vi "robot_position.vi"(10 "Distance Along Arc":u16, 11 "Wheel Angle":i8) -> (1 "New X Position":i16, 2 "New Y Position":i16, 3 "Turning Radius":u8)   [LabVIEW 2009]
uses:
  <vilib>/Platform/TimedLoop/XDataNode/XDataNode.xnode
  <vilib>/Platform/TimedLoop/XDataNode/loadlvalarms.vi
  <vilib>/Platform/TimedLoop/XDataNode/timing_clust.ctl
  <vilib>/Platform/TimedLoop/XDataNode/nitl_modes.ctl
  <vilib>/Platform/TimedLoop/XDataNode/wakeup.ctl
  <vilib>/Platform/TimedLoop/XDataNode/XDNodeRunTimeDep.lvlib
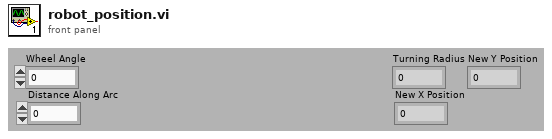
[diagram p1: front panel]
types:
  T1 = typedef "XDNodeRunTimeDep.lvlib/timing_clust.ctl" = cluster{"Expected End [f-1]":u64, "Actual End [f-1]":u64, "Finished Late? [f-1]":bool, "Expected End [i-1]":u64, "Actual End [i-1]":u64, "Finished Late? [i-1]":bool, "Expected Start [i]":u64, "Actual Start [i]":u64, "Expected Start [f]":u64, "Actual Start [f]":u64, "Source Name":string, "Structure Name":string, "Period":i64, "Deadline":i64, "Offset":i64, "Start":i64, "Priority":i32, "Timeout":i32, "Mode":T2, "Wakeup Reason":T3, "Error":errorcluster, "Source Type":string, "Secondary Source Type":string, "Global End Time":u64, "Global Start Time":u64, "Frame Duration":u64, "Iteration Duration":u64, "Assigned CPU":i32, "I/O Scan Engine Mode":u32}
  T2 = typedef "XDNodeRunTimeDep.lvlib/nitl_modes.ctl" = enum32{"No Change", "Process missed periods, maintain original phase", "Discard missed periods, maintain original phase", "Process missed periods, ignore original phase", "Discard missed periods, ignore original phase"}
  T3 = typedef "XDNodeRunTimeDep.lvlib/wakeup.ctl" = enum32{"Normal", "Aborted", "Asynchronous wakeup", "Timing source error", "Timed loop error", "Timeout"}
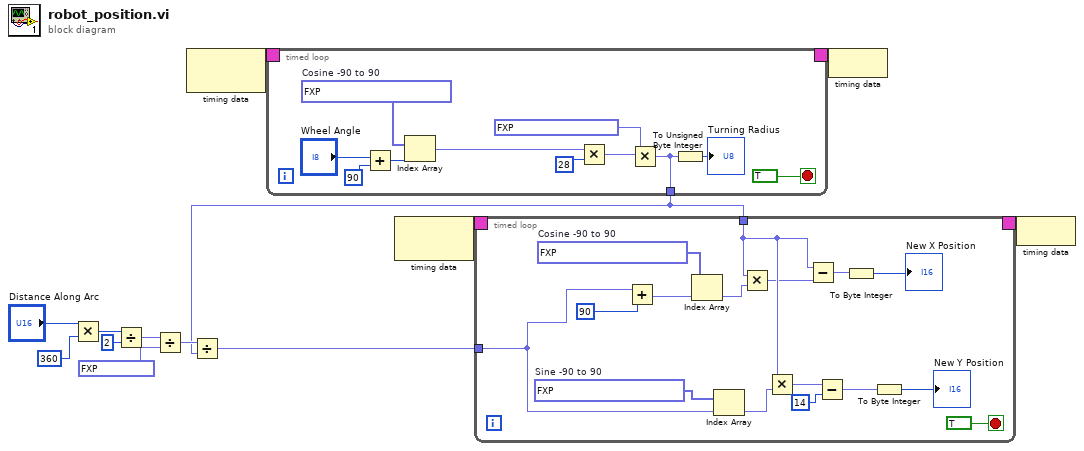
[diagram p0: block diagram]
diagram:
  n1 = Multiply(x="Distance Along Arc", y=u16 360) -> (x*y=w11:u16)
  n2 = Divide(x=w11, y=u8 2) -> (x/y=w6:fxp<+/-,32,16>)
  n3 = Divide(x=w6, y=fxp<+,12,2> 3.1416015625) -> (x/y=w8:fxp<+/-,33,15>)
  n4 = node-c288() -> (w5:T1)  [unwired: 1 in]
  n5 = timed-loop {
    timing: w5 -> [_]
    timing-out: [_] -> w4
    tunnel: [w24] -> w1
    stop <- TRUE stop-if-true
    w22 = fxp<+/-,16,1>[] [0.0, 0.0174560546875, 0.034912109375, 0.052337646484375, 0.06976318359375, 0.087158203125, 0.104522705078125, 0.121856689453125, 0.13916015625, 0.15643310546875, 0.17364501953125, 0.1907958984375, 0.207916259765625, 0.224945068359375, 0.241912841796875, 0.258819580078125, 0.275634765625, 0.2923583984375, 0.30902099609375, 0.3255615234375, 0.342010498046875, 0.358367919921875, 0.374603271484375, 0.390716552734375, 0.40673828125, 0.422607421875, 0.438385009765625, 0.4539794921875, 0.469482421875, 0.48480224609375, 0.5, 0.515045166015625, 0.5299072265625, 0.544647216796875, 0.5592041015625, 0.573577880859375, 0.587799072265625, 0.601806640625, 0.61566162109375, 0.62933349609375, 0.642791748046875, 0.65606689453125, 0.66912841796875, 0.6820068359375, 0.694671630859375, 0.70709228515625, 0.719329833984375, 0.731353759765625, 0.743133544921875, 0.75469970703125, 0.76605224609375, 0.77716064453125, 0.78802490234375, 0.79864501953125, 0.80902099609375, 0.81915283203125, 0.82904052734375, 0.83868408203125, 0.848052978515625, 0.857177734375, 0.86602783203125, 0.8746337890625, 0.8829345703125, 0.891021728515625, 0.8988037109375, 0.90631103515625, 0.913543701171875, 0.920501708984375, 0.92718505859375, 0.93359375, 0.939697265625, 0.945526123046875, 0.9510498046875, 0.956298828125, 0.961273193359375, 0.965911865234375, 0.970306396484375, 0.974365234375, 0.9781494140625, 0.98162841796875, 0.98480224609375, 0.987701416015625, 0.990264892578125, 0.9925537109375, 0.9945068359375, 0.996185302734375, 0.99755859375, 0.998626708984375, 0.9993896484375, 0.999847412109375, 0.999969482421875, 0.999847412109375, 0.9993896484375, 0.998626708984375, 0.99755859375, 0.996185302734375, 0.9945068359375, 0.9925537109375, 0.990264892578125, 0.987701416015625, 0.98480224609375, 0.98162841796875, 0.9781494140625, 0.974365234375, 0.970306396484375, 0.965911865234375, 0.961273193359375, 0.956298828125, 0.9510498046875, 0.945526123046875, 0.939697265625, 0.93359375, 0.92718505859375, 0.920501708984375, 0.913543701171875, 0.90631103515625, 0.8988037109375, 0.891021728515625, 0.8829345703125, 0.8746337890625, 0.86602783203125, 0.857177734375, 0.848052978515625, 0.83868408203125, 0.82904052734375, 0.81915283203125, 0.80902099609375, 0.79864501953125, 0.78802490234375, 0.77716064453125, 0.76605224609375, 0.75469970703125, 0.743133544921875, 0.731353759765625, 0.719329833984375, 0.70709228515625, 0.694671630859375, 0.6820068359375, 0.66912841796875, 0.65606689453125, 0.642791748046875, 0.62933349609375, 0.61566162109375, 0.601806640625, 0.587799072265625, 0.573577880859375, 0.5592041015625, 0.544647216796875, 0.5299072265625, 0.515045166015625, 0.5, 0.48480224609375, 0.469482421875, 0.4539794921875, 0.438385009765625, 0.422607421875, 0.40673828125, 0.390716552734375, 0.374603271484375, 0.358367919921875, 0.342010498046875, 0.3255615234375, 0.30902099609375, 0.2923583984375, 0.275634765625, 0.258819580078125, 0.241912841796875, 0.224945068359375, 0.207916259765625, 0.1907958984375, 0.17364501953125, 0.15643310546875, 0.13916015625, 0.121856689453125, 0.104522705078125, 0.087158203125, 0.06976318359375, 0.052337646484375, 0.034912109375, 0.0174560546875, 0.0]  # Cosine -90 to 90
    n6 = Add(x="Wheel Angle", y=i8 90) -> (x+y=w18:i8)
    n7 = Index Array(array=w22, index=w18) -> (element=w21:fxp<+/-,16,1>)
    n8 = Multiply(x=w21, y=i8 28) -> (x*y=w23:fxp<+/-,24,9>)
    n9 = Multiply(x=w23, y=fxp<+/-,24,9> 3.1416015625) -> (x*y=w24:fxp<+/-,46,16>)
    n10 = To Unsigned Byte Integer(number=w24) -> (unsigned 8bit integer=→"Turning Radius":u8)
  }
  n11 = Divide(x=w8, y=w1) -> (x/y=w7:fxp<+/-,64,45>)
  n12 = node-c288() -> (w3:T1)  [unwired: 1 in]
  n13 = timed-loop {
    timing: w3 -> [_]
    timing-out: [_] -> w2
    tunnel: w7 -> [w42]
    tunnel: w1 -> [w41]
    stop <- TRUE stop-if-true
    w38 = fxp<+/-,16,1>[] [0.0, 0.0174560546875, 0.034912109375, 0.052337646484375, 0.06976318359375, 0.087158203125, 0.104522705078125, 0.121856689453125, 0.13916015625, 0.15643310546875, 0.17364501953125, 0.1907958984375, 0.207916259765625, 0.224945068359375, 0.241912841796875, 0.258819580078125, 0.275634765625, 0.2923583984375, 0.30902099609375, 0.3255615234375, 0.342010498046875, 0.358367919921875, 0.374603271484375, 0.390716552734375, 0.40673828125, 0.422607421875, 0.438385009765625, 0.4539794921875, 0.469482421875, 0.48480224609375, 0.5, 0.515045166015625, 0.5299072265625, 0.544647216796875, 0.5592041015625, 0.573577880859375, 0.587799072265625, 0.601806640625, 0.61566162109375, 0.62933349609375, 0.642791748046875, 0.65606689453125, 0.66912841796875, 0.6820068359375, 0.694671630859375, 0.70709228515625, 0.719329833984375, 0.731353759765625, 0.743133544921875, 0.75469970703125, 0.76605224609375, 0.77716064453125, 0.78802490234375, 0.79864501953125, 0.80902099609375, 0.81915283203125, 0.82904052734375, 0.83868408203125, 0.848052978515625, 0.857177734375, 0.86602783203125, 0.8746337890625, 0.8829345703125, 0.891021728515625, 0.8988037109375, 0.90631103515625, 0.913543701171875, 0.920501708984375, 0.92718505859375, 0.93359375, 0.939697265625, 0.945526123046875, 0.9510498046875, 0.956298828125, 0.961273193359375, 0.965911865234375, 0.970306396484375, 0.974365234375, 0.9781494140625, 0.98162841796875, 0.98480224609375, 0.987701416015625, 0.990264892578125, 0.9925537109375, 0.9945068359375, 0.996185302734375, 0.99755859375, 0.998626708984375, 0.9993896484375, 0.999847412109375, 0.999969482421875, 0.999847412109375, 0.9993896484375, 0.998626708984375, 0.99755859375, 0.996185302734375, 0.9945068359375, 0.9925537109375, 0.990264892578125, 0.987701416015625, 0.98480224609375, 0.98162841796875, 0.9781494140625, 0.974365234375, 0.970306396484375, 0.965911865234375, 0.961273193359375, 0.956298828125, 0.9510498046875, 0.945526123046875, 0.939697265625, 0.93359375, 0.92718505859375, 0.920501708984375, 0.913543701171875, 0.90631103515625, 0.8988037109375, 0.891021728515625, 0.8829345703125, 0.8746337890625, 0.86602783203125, 0.857177734375, 0.848052978515625, 0.83868408203125, 0.82904052734375, 0.81915283203125, 0.80902099609375, 0.79864501953125, 0.78802490234375, 0.77716064453125, 0.76605224609375, 0.75469970703125, 0.743133544921875, 0.731353759765625, 0.719329833984375, 0.70709228515625, 0.694671630859375, 0.6820068359375, 0.66912841796875, 0.65606689453125, 0.642791748046875, 0.62933349609375, 0.61566162109375, 0.601806640625, 0.587799072265625, 0.573577880859375, 0.5592041015625, 0.544647216796875, 0.5299072265625, 0.515045166015625, 0.5, 0.48480224609375, 0.469482421875, 0.4539794921875, 0.438385009765625, 0.422607421875, 0.40673828125, 0.390716552734375, 0.374603271484375, 0.358367919921875, 0.342010498046875, 0.3255615234375, 0.30902099609375, 0.2923583984375, 0.275634765625, 0.258819580078125, 0.241912841796875, 0.224945068359375, 0.207916259765625, 0.1907958984375, 0.17364501953125, 0.15643310546875, 0.13916015625, 0.121856689453125, 0.104522705078125, 0.087158203125, 0.06976318359375, 0.052337646484375, 0.034912109375, 0.0174560546875, 0.0]  # Cosine -90 to 90
    w35 = fxp<+/-,16,1>[] [-1.0, -0.999847412109375, -0.9993896484375, -0.998626708984375, -0.99755859375, -0.996185302734375, -0.9945068359375, -0.9925537109375, -0.990264892578125, -0.987701416015625, -0.98480224609375, -0.98162841796875, -0.9781494140625, -0.974365234375, -0.970306396484375, -0.965911865234375, -0.961273193359375, -0.956298828125, -0.9510498046875, -0.945526123046875, -0.939697265625, -0.93359375, -0.92718505859375, -0.920501708984375, -0.913543701171875, -0.90631103515625, -0.8988037109375, -0.891021728515625, -0.8829345703125, -0.8746337890625, -0.86602783203125, -0.857177734375, -0.848052978515625, -0.83868408203125, -0.82904052734375, -0.81915283203125, -0.80902099609375, -0.79864501953125, -0.78802490234375, -0.77716064453125, -0.76605224609375, -0.75469970703125, -0.743133544921875, -0.731353759765625, -0.719329833984375, -0.70709228515625, -0.694671630859375, -0.6820068359375, -0.66912841796875, -0.65606689453125, -0.642791748046875, -0.62933349609375, -0.61566162109375, -0.601806640625, -0.587799072265625, -0.573577880859375, -0.5592041015625, -0.544647216796875, -0.5299072265625, -0.515045166015625, -0.5, -0.48480224609375, -0.469482421875, -0.4539794921875, -0.438385009765625, -0.422607421875, -0.40673828125, -0.390716552734375, -0.374603271484375, -0.358367919921875, -0.342010498046875, -0.3255615234375, -0.30902099609375, -0.2923583984375, -0.275634765625, -0.258819580078125, -0.241912841796875, -0.224945068359375, -0.207916259765625, -0.1907958984375, -0.17364501953125, -0.15643310546875, -0.13916015625, -0.121856689453125, -0.104522705078125, -0.087158203125, -0.06976318359375, -0.052337646484375, -0.034912109375, -0.0174560546875, 0.0, 0.0174560546875, 0.034912109375, 0.052337646484375, 0.06976318359375, 0.087158203125, 0.104522705078125, 0.121856689453125, 0.13916015625, 0.15643310546875, 0.17364501953125, 0.1907958984375, 0.207916259765625, 0.224945068359375, 0.241912841796875, 0.258819580078125, 0.275634765625, 0.2923583984375, 0.30902099609375, 0.3255615234375, 0.342010498046875, 0.358367919921875, 0.374603271484375, 0.390716552734375, 0.40673828125, 0.422607421875, 0.438385009765625, 0.4539794921875, 0.469482421875, 0.48480224609375, 0.5, 0.515045166015625, 0.5299072265625, 0.544647216796875, 0.5592041015625, 0.573577880859375, 0.587799072265625, 0.601806640625, 0.61566162109375, 0.62933349609375, 0.642791748046875, 0.65606689453125, 0.66912841796875, 0.6820068359375, 0.694671630859375, 0.70709228515625, 0.719329833984375, 0.731353759765625, 0.743133544921875, 0.75469970703125, 0.76605224609375, 0.77716064453125, 0.78802490234375, 0.79864501953125, 0.80902099609375, 0.81915283203125, 0.82904052734375, 0.83868408203125, 0.848052978515625, 0.857177734375, 0.86602783203125, 0.8746337890625, 0.8829345703125, 0.891021728515625, 0.8988037109375, 0.90631103515625, 0.913543701171875, 0.920501708984375, 0.92718505859375, 0.93359375, 0.939697265625, 0.945526123046875, 0.9510498046875, 0.956298828125, 0.961273193359375, 0.965911865234375, 0.970306396484375, 0.974365234375, 0.9781494140625, 0.98162841796875, 0.98480224609375, 0.987701416015625, 0.990264892578125, 0.9925537109375, 0.9945068359375, 0.996185302734375, 0.99755859375, 0.998626708984375, 0.9993896484375, 0.999847412109375, 0.999969482421875]  # Sine -90 to 90
    n14 = Add(x=w42, y=u16 90) -> (x+y=w39:fxp<+/-,64,46>)
    n15 = Index Array(array=w38, index=w39) -> (element=w37:fxp<+/-,16,1>)
    n16 = Index Array(array=w35, index=w42) -> (element=w34:fxp<+/-,16,1>)
    n17 = Multiply(x=w41, y=w37) -> (x*y=w36:fxp<+/-,60,15>)
    n18 = Multiply(x=w41, y=w34) -> (x*y=w33:fxp<+/-,60,15>)
    n19 = Subtract(x=w41, y=w36) -> (x-y=w31:fxp<+/-,62,17>)
    n20 = Subtract(x=w33, y=i8 14) -> (x-y=w29:fxp<+/-,61,16>)
    n21 = To Byte Integer(number=w31) -> (8bit integer=→"New X Position":i8)
    n22 = To Byte Integer(number=w29) -> (8bit integer=→"New Y Position":i8)
  }
  n23 = node-c288(w4) -> ()
  n24 = node-c288(w2) -> ()
